vi "Speed LUT.vi"(10 "LUT speed":dbl[][](array[numeric]), 11 "Speed":dbl) -> (3 "Motor Speed index":dbl)   [LabVIEW 2020, in "Hiden Scanner.lvlib"]
uses:
  Hiden Scanner.lvlib
  <vilib>/gmath/NI_Gmath.lvlib
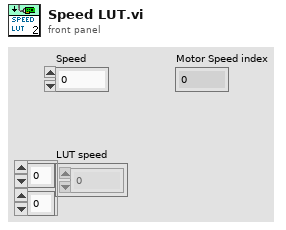
[diagram p1: front panel]
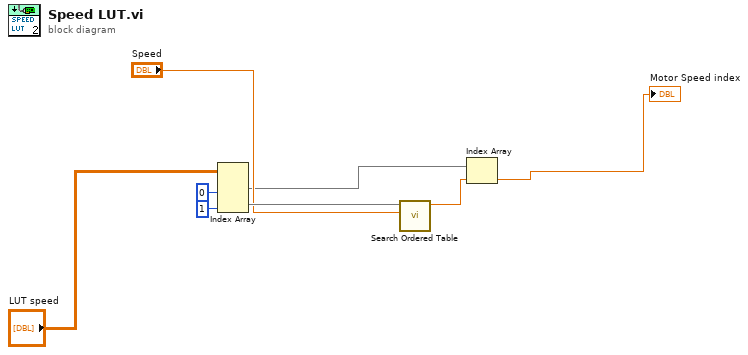
[diagram p0: block diagram]
diagram:
  n1 = Index Array(array="LUT speed", index (col) #1=0 ("disabled index (col)"), index (col) #2=1 ("index (col)")) -> (element #1=w4:dbl[], element #2=w6:dbl[])  [unwired: 2 in]
  n2 = call <vilib>:"Search Ordered Table.vi"("x value"="Speed", "ordered x array"=w6) -> ("fractional index"=w3:dbl)  [unwired: 9 in]
  n3 = Index Array(array=w4, index=w3) -> (element=→"Motor Speed index":dbl)
